vi "Global 1.vi"() -> ()   [LabVIEW 2025]
panel:
  in  "Start":bool
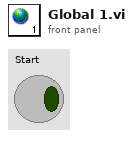
[diagram p1: front panel]
diagram:
